vi "Toggle OCP.vi"(8 "error in":errorcluster, 10 "Toggle(F:OFF)":bool, 11 "Modbus instance in":refnum<class "Modbus API.lvclass">) -> (0 "error out":errorcluster, 3 "Modbus instance out":refnum<class "Modbus API.lvclass">)   [LabVIEW 2025, in "Hanmatek HM310T.lvlib"]
uses:
  <vilib>/NI/Modbus Library/API/Modbus API.lvclass
  f8f31601-b21c-4c8d-ab26-724c93e45244.vi
  <instrlib>/Hanmatek HM310T/Hanmatek HM310T.lvlib
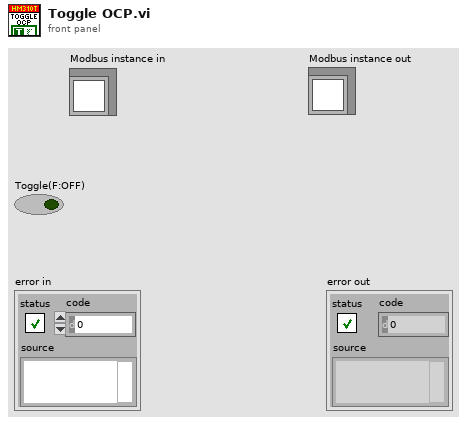
[diagram p1: front panel]
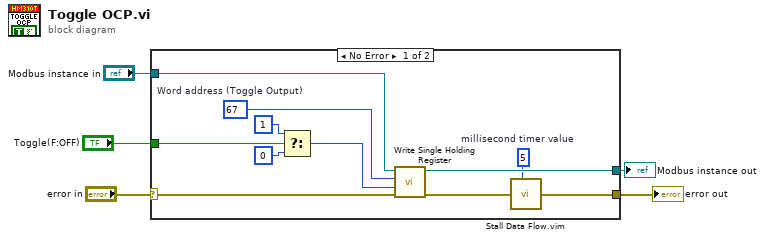
[diagram p0: block diagram]
diagram:
  n1 = case shown="No Error" "error in" {
    selector: "error in" -> [w10 w18]
    tunnel: [w8 w18] -> w5
    tunnel: "Toggle(F:OFF)" -> [w14 _]
    tunnel: [w9 w17] -> w2
    tunnel: "Modbus instance in" -> [w6 w17]
    frame No Error {
      w7 = u32 5  # millisecond timer value
      w15 = u16 67  # Word address (Toggle Output)
      n2 = Select(t=u16 1 ("Word (0)"), s=w14, f=u16 0 ("Word (0)")) -> (s? t:f=w11:u16)
      n3 = call-dynamic "Write Single Holding Register.vi"("error in"=w10, "register to write"=w11, "address"=w15, "Modbus instance in"=w6) -> ("error out"=w16:errorcluster, "Modbus instance out"=w9:refnum<class "Modbus API.lvclass">)  [unwired: 6 in]
      n4 = call "Stall Data Flow.vim"("value in"=w16, "milliseconds to wait"=w7) -> ("value out"=w8:errorcluster)  [unwired: 1 out]
    }
    frame Error {
    }
  }
  "error out" <- w5
  "Modbus instance out" <- w2
